vi "ADA do.vi"(0 "Data in":T1={"[V]"=0.0, "Vertical sum"=0.0, "Horizontal sum"=0.0, "auto Loopback"=FALSE, "Auto Balance"=FALSE, "Out Cmd"=0, "Motor Cmd"=0, "ADC Values"=[], "Clouds ctrl"=FALSE, "Cloud Det"=FALSE, "Cloud Sens"=0, "Loops"=0, "VISA res"="COM3"}, 1 "Auto diode":bool, 5 "ADA  level 1 [V] in":dbl, 7 "ADA  level 2 [V] in":dbl, 9 "ADA  level 3 [V] in":dbl, 11 "Speed Control in":u8, 12 "Loopback":bool) -> (3 "ADA off request":bool, 4 "Data out":T1={"[V]"=0.0, "Vertical sum"=0.0, "Horizontal sum"=0.0, "auto Loopback"=FALSE, "Auto Balance"=FALSE, "Out Cmd"=0, "Motor Cmd"=0, "ADC Values"=[], "Clouds ctrl"=FALSE, "Cloud Det"=FALSE, "Cloud Sens"=0, "Loops"=0, "VISA res"="COM3"}, 6 "ADA  level 1 [V]":dbl, 8 "ADA  level 2 [V]":dbl, 10 "ADA  level 3 [V]":dbl, 15 "Speed Control out":u8)   [LabVIEW 2014]
uses:
  Ctrls/Data cluster.ctl
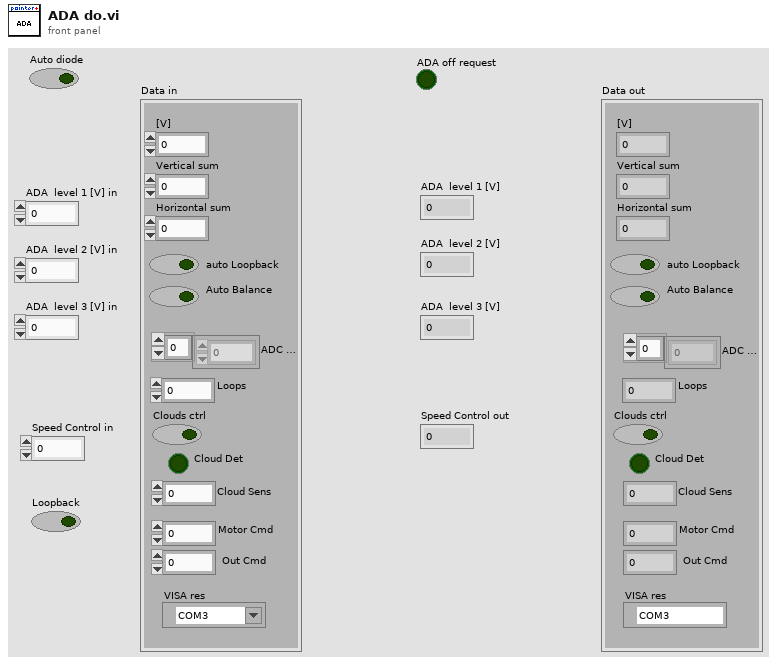
[diagram p1: front panel]
types:
  T1 = typedef "Data cluster.ctl" = cluster{"[V]":dbl, "Vertical sum":dbl, "Horizontal sum":dbl, "auto Loopback":bool, "Auto Balance":bool, "Out Cmd":i32, "Motor Cmd":i32, "ADC Values":dbl[], "Clouds ctrl":bool, "Cloud Det":bool, "Cloud Sens":i8, "Loops":u8, "VISA res":refnum<visa-resource-name>}
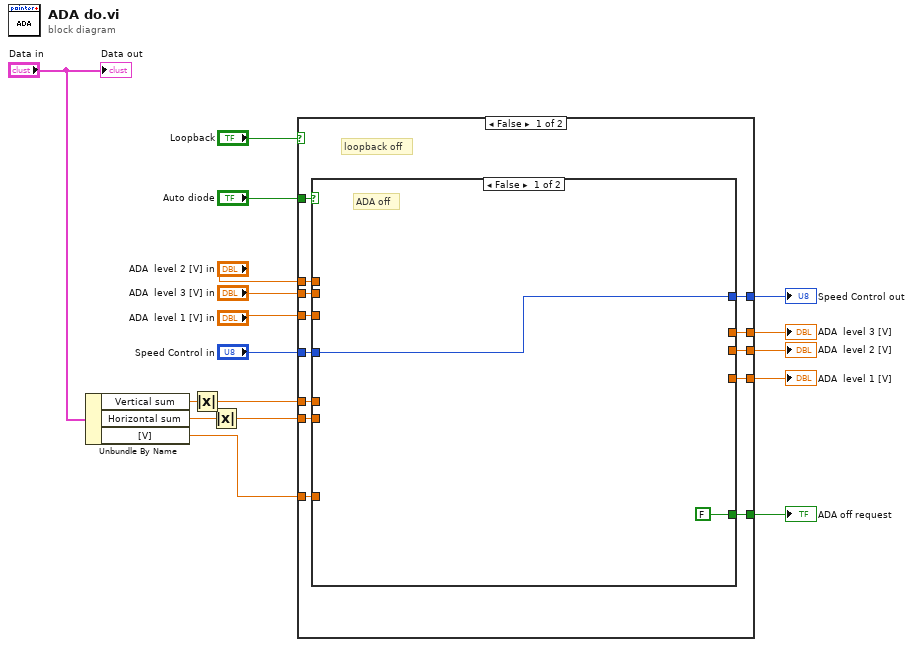
[diagram p0: block diagram]
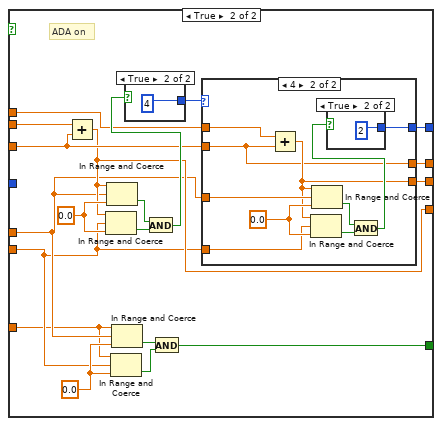
[diagram p2: hidden frame]
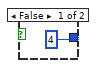
[diagram p4: hidden frame]
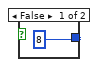
[diagram p5: hidden frame]
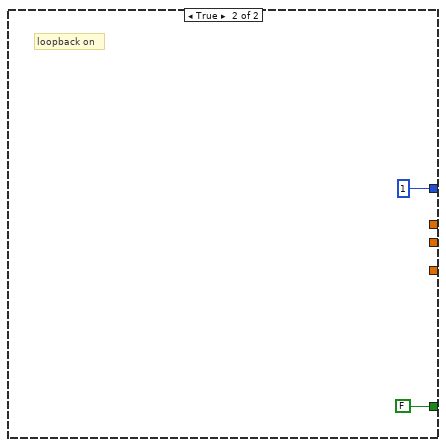
[diagram p6: hidden frame]
diagram:
  n1 = Unbundle By Name("Data in") -> ("Vertical sum"=w8:dbl, "Horizontal sum"=w6:dbl, "[V]"=w3:dbl)
  n2 = Absolute Value(x=w8) -> (abs(x)=w7:dbl)
  n3 = Absolute Value(x=w6) -> (abs(x)=w5:dbl)
  n4 = case shown="False" "Loopback" {
    tunnel: [w28 u8 1 ("Speed Control")] -> w9
    tunnel: "Speed Control in" -> [w29 _]
    tunnel: "Auto diode" -> [w30 _]
    tunnel: w7 -> [w27 _]
    tunnel: w5 -> [w26 _]
    tunnel: "ADA  level 3 [V] in" -> [w25 _]
    tunnel: "ADA  level 1 [V] in" -> [w24 _]
    tunnel: "ADA  level 2 [V] in" -> [w23 _]
    tunnel: [w22 _] -> w15
    tunnel: [w21 _] -> w16
    tunnel: [w20 _] -> w17
    tunnel: w3 -> [w19 _]
    tunnel: [w18 FALSE] -> w2
    frame False {
      # "loopback off"
      n5 = case shown="False" w30 {
        tunnel: [w32 w47] -> w28
        tunnel: w29 -> [w32 _]
        tunnel: w27 -> [_ w36]
        tunnel: w26 -> [_ w35]
        tunnel: w25 -> [_ w45]
        tunnel: w24 -> [_ w44]
        tunnel: w23 -> [_ w43]
        tunnel: [_ w42] -> w22
        tunnel: [_ w41] -> w21
        tunnel: [_ w40] -> w20
        tunnel: w19 -> [_ w34]
        tunnel: [FALSE w33] -> w18
        frame False {
          # "ADA off"
        }
        frame True {
          w39 = 0.0 ("upper limit")
          w49 = 0.0 ("upper limit")
          # "ADA on"
          n6 = Add(x=w45, y=w44) -> (x+y=w40:dbl)
          n7 = In Range and Coerce(upper limit=w40, x=w35, lower limit=w49) -> (In Range?=w50:bool)  [unwired: 1 out]
          n8 = In Range and Coerce(upper limit=w40, x=w36, lower limit=w49) -> (In Range?=w51:bool)  [unwired: 1 out]
          n9 = In Range and Coerce(upper limit=w34, x=w35, lower limit=w39) -> (In Range?=w38:bool)  [unwired: 1 out]
          n10 = In Range and Coerce(upper limit=w34, x=w36, lower limit=w39) -> (In Range?=w37:bool)  [unwired: 1 out]
          n11 = And(x=w51, y=w50) -> (x .and. y?=w46:bool)
          n12 = case shown="True" w46 {
            tunnel: [u8 8 ("Speed Control") u8 4 ("Speed Control")] -> w48
            frame False {
            }
            frame True {
            }
          }
          n13 = And(x=w37, y=w38) -> (x .and. y?=w33:bool)
          n14 = case shown="4" w48 {
            selector: w48 -> [w52 _]
            tunnel: [w52 w59] -> w47
            tunnel: w44 -> [_ w53]
            tunnel: w35 -> [_ w57]
            tunnel: w36 -> [_ w56]
            tunnel: w43 -> [_ w55]
            tunnel: [_ w54] -> w42
            tunnel: [_ w53] -> w41
            frame 8, Default {
            }
            frame 4 {
              w60 = 0.0 ("upper limit")
              n15 = Add(x=w55, y=w53) -> (x+y=w54:dbl)
              n16 = In Range and Coerce(upper limit=w54, x=w57, lower limit=w60) -> (In Range?=w61:bool)  [unwired: 1 out]
              n17 = In Range and Coerce(upper limit=w54, x=w56, lower limit=w60) -> (In Range?=w62:bool)  [unwired: 1 out]
              n18 = And(x=w62, y=w61) -> (x .and. y?=w58:bool)
              n19 = case shown="True" w58 {
                tunnel: [u8 4 ("Speed Control") u8 2 ("Speed Control")] -> w59
                frame False {
                }
                frame True {
                }
              }
            }
          }
        }
      }
    }
    frame True {
      # "loopback on"
    }
  }
  "ADA  level 1 [V]" <- w17
  "ADA  level 3 [V]" <- w16
  "ADA  level 2 [V]" <- w15
  "Speed Control out" <- w9
  "ADA off request" <- w2
  "Data out" <- "Data in"
